vi "hpcnc move to origin.vi"(8 "error in (no error)":errorcluster, 9 "Speed":i32=1000, 11 "VISA Refnum in":refnum<visa-resource-name>) -> ()   [LabVIEW 2014]
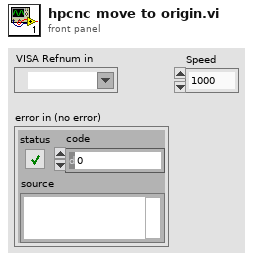
[diagram p1: front panel]
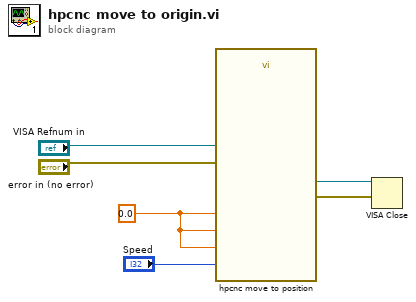
[diagram p0: block diagram]
diagram:
  w4 = 0.0 ("X")
  n1 = call "hpcnc move to position.vi"("VISA Refnum in"="VISA Refnum in", "X"=w4, "Y"=w4, "Z"=w4, "Speed"="Speed", "error in"="error in (no error)") -> ("VISA Refnum out"=w6:refnum<visa-resource-name>, "error out"=w5:errorcluster)  [unwired: 12 in]
  n2 = VISA Close(VISA resource name=w6, error in (no error)=w5) -> ()  [unwired: 1 out]
